vi "CalData to EEPROM.vi"(11 "Array 4":dbl[][](array[numeric])) -> (1 "Array 2":dbl[](array[numeric]), 2 "Array":dbl[][](array[numeric]), 3 "Array 3":dbl[](array[numeric]))   [LabVIEW 2013]
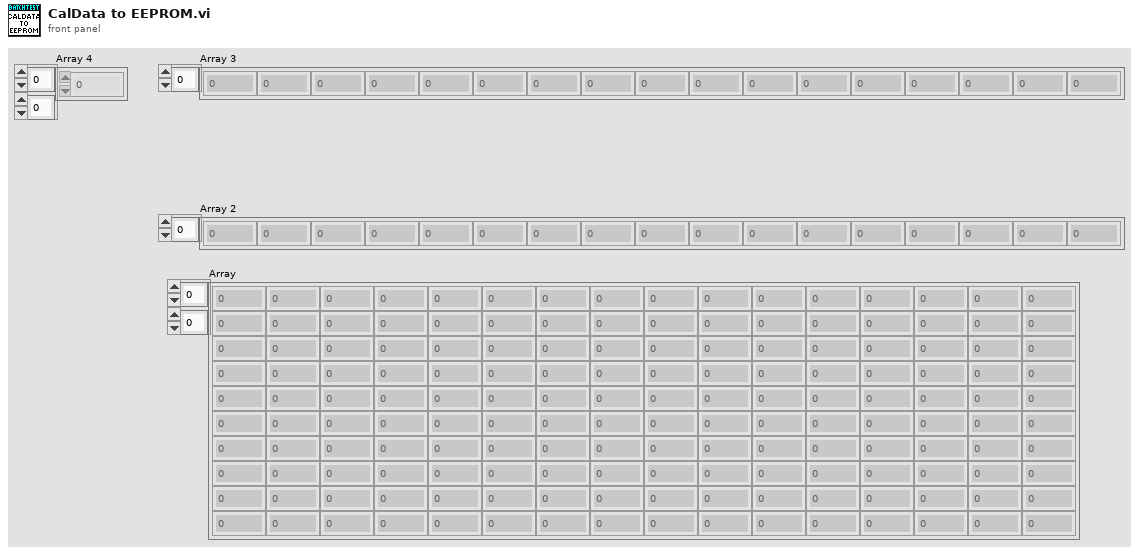
[diagram p1: front panel]
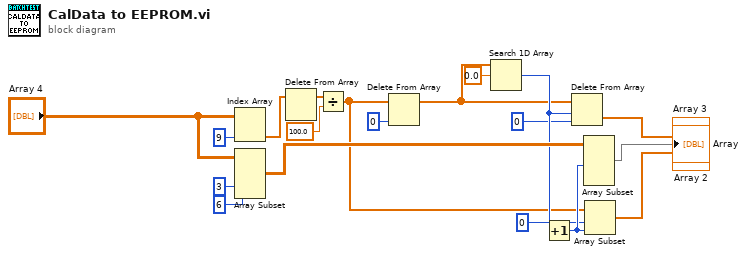
[diagram p0: block diagram]
diagram:
  n1 = Index Array(array="Array 4", index (col)=9 ("disabled index (col)")) -> (element=w5:dbl[])  [unwired: 1 in]
  n2 = Array Subset(array="Array 4", index (col)=3 ("index"), length (col)=6 ("length")) -> (w17:dbl[][])  [unwired: 2 in]
  n3 = Delete From Array(array=w5) -> (array with subset deleted=w6:dbl[])  [unwired: 2 in, 1 out]
  n4 = Divide(x=w6, y=100.0) -> (x/y=w13:dbl[])
  n5 = Delete From Array(array=w13, index=0) -> (array with subset deleted=w11:dbl[])  [unwired: 1 in, 1 out]
  n6 = Search 1D Array(1D array=w11, element=0.0) -> (index of element=w14:i32)  [unwired: 1 in]
  n7 = Increment(x=w14) -> (x+1=w19:i32)
  n8 = Delete From Array(array=w11, length=w14, index=0) -> (deleted portion=→"Array 3":dbl[])  [unwired: 1 out]
  n9 = Array Subset(array=w17, length (row)=w19) -> (→"Array":dbl[][])  [unwired: 3 in]
  n10 = Array Subset(array=w13, index=0, length=w19) -> (→"Array 2":dbl[])
